vi "Register UI user events.vi"(8 "error in (no error)":errorcluster, 11 "Execution UI In":refnum<class "Execution UI.lvclass">) -> (0 "error out":errorcluster, 2 "output cluster":T1, 3 "Execution UI Out":refnum<class "Execution UI.lvclass">)   [LabVIEW 2020, in "Execution UI.lvclass"]
uses:
  Execution UI.lvclass
  Result Classes/Method Result/Method Result.lvclass
  Result Classes/Test Case Result/Test Case Result.lvclass
  Result Classes/Test Suite Result/Test Suite Result.lvclass
  Execution UI.lvclass/Execution UI.ctl
  Result Collector/Result Collector.lvclass
  Test Runner/Test Runner.lvclass
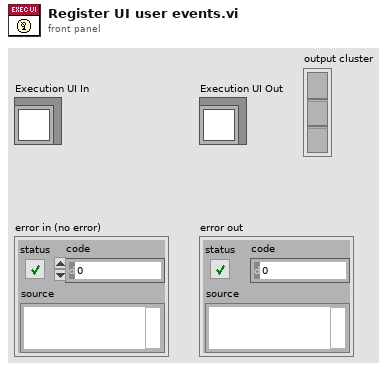
[diagram p1: front panel]
types:
  T1 = cluster{"Event Registration Refnum":refnum<event-registration>, "Event Registration Refnum":refnum<event-registration>, "Event Registration Refnum":refnum<event-registration>}
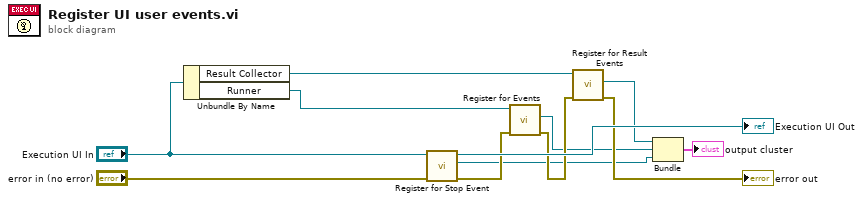
[diagram p0: block diagram]
diagram:
  n1 = Unbundle By Name("Execution UI In") -> ("Result Collector"=w12:refnum<class "Result Collector.lvclass">, "Runner"=w6:refnum<class "Test Runner.lvclass">)
  n2 = call "Register for Stop Event.vi"("error in (no error)"="error in (no error)", "Execution UI In"="Execution UI In") -> ("error out"=w5:errorcluster, "Event Registration Refnum"=w3:refnum<event-registration>, "Execution UI Out"=→"Execution UI Out":refnum<class "Execution UI.lvclass">)  [unwired: 7 in]
  n3 = call "Register for Events.vi"("error in (no error)"=w5, "Test Runner In"=w6) -> ("error out"=w4:errorcluster, "Event Registration Refnum"=w2:refnum<event-registration>)  [unwired: 7 in, 1 out]
  n4 = call "Register for Result Events.vi"("error in (no error)"=w4, "Result Collector In"=w12) -> ("error out"=→"error out":errorcluster, "Event Registration Refnum"=w9:refnum<event-registration>)  [unwired: 7 in, 1 out]
  n5 = Bundle("Event Registration Refnum"=w9, "Event Registration Refnum"=w2, "Event Registration Refnum"=w3) -> (→"output cluster":T1)  [unwired: 1 in]
